vi "LVClass_HasoEngine Get AlgoType.vi"(0 "HasoEngine in":refnum<class "HasoEngine.lvclass">, 11 "error in (no error)":errorcluster) -> (4 "HasoEngine out":refnum<class "HasoEngine.lvclass">, 6 "algo_type":i32, 15 "error out":errorcluster)   [LabVIEW 2020, in "HasoEngine.lvclass"]
doc: "Spots detection algorithm type getter.\n\n--------------------------------------------------------------------------------\n\n<B>HasoEngineIn </B> : HasoEngine object.\n<B>HasoEngineOut </B> : HasoEngine object.\n<B>algo_type </B> : Spots detection algorithm type : standard (0) or fast (1).\n<B>ErrorIn </B> : Error\n<B>ErrorOut </B> : Error\n\n--------------------------------------------------------------------------------"
uses:
  HasoEngine.lvclass
  HasoEngine.lvclass/HasoEngine.ctl
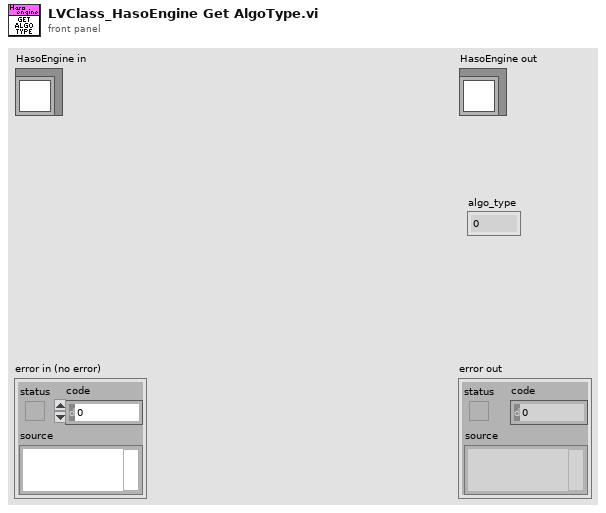
[diagram p1: front panel]
types:
  T1 = typedef "ClassID.ctl" = i64
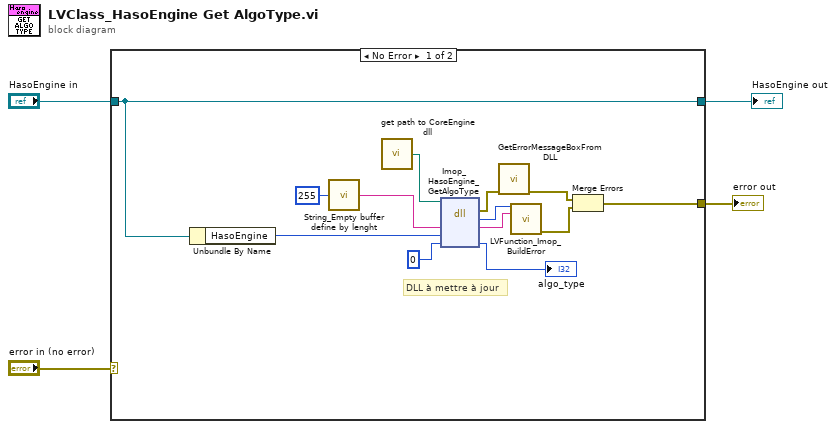
[diagram p0: block diagram]
diagram:
  n1 = case shown="No Error" "error in (no error)" {
    selector: "error in (no error)" -> [_ w18]
    tunnel: "HasoEngine in" -> [w12 w19]
    tunnel: [w12 w19] -> w1
    tunnel: [w7 w18] -> w2
    frame No Error {
      # "DLL à mettre à jour"
      n2 = Unbundle By Name(w12) -> ("HasoEngine"=w11:T1)
      n3 = call "String_Empty buffer define by lenght.vi"("Lenght (255)"=255) -> ("Empty buffer"=w15:string)
      n4 = call "get path to CoreEngine dll.vi"() -> ("path to wavekit library"=w14:path)  [unwired: 14 in, 1 out]
      n5 = dll-call lib="D:/soft/HASO_v3/SVN_trunk/ImOpCoreEngine4_LV2011/DLLs/c_interface_vc100.dll" fn="Imop_HasoEngine_GetAlgoType"(path in=w14, "message"=w15, "hasoEngine"=w11, "algo_type"=0) -> (error out=w13:errorcluster, "return type"=w16:i32, "message"=w17:string, "algo_type"=→"algo_type":i32)  [unwired: 3 in, 1 out]
      n6 = call "GetErrorMessageBoxFromDLL.vi"("error IN"=w13) -> ("error OUT"=w9:errorcluster)  [unwired: 10 in]
      n7 = call "LVFunction_Imop_BuildError.vi"("code"=w16, "String to Prepend to source (\"\")"=w17) -> ("error out"=w8:errorcluster)  [unwired: 13 in]
      n8 = Merge Errors(w9, w8) -> (w7:errorcluster)
    }
    frame Error {
    }
  }
  "error out" <- w2
  "HasoEngine out" <- w1
